vi "Common_Py_Get_Diff_Stats.vi"(0 "session in":refnum<k35>, 5 "module path":path=path "D:/dev/Guy_Storage/Work/Cancun/MW_Display_Test/Magewell Capture/Capture_LV.py", 11 "error in":errorcluster) -> (4 "session out":refnum<k35>, 6 "module path out":path, 14 "Diff_Stats":T1, 15 "error out":errorcluster)   [LabVIEW 2023]
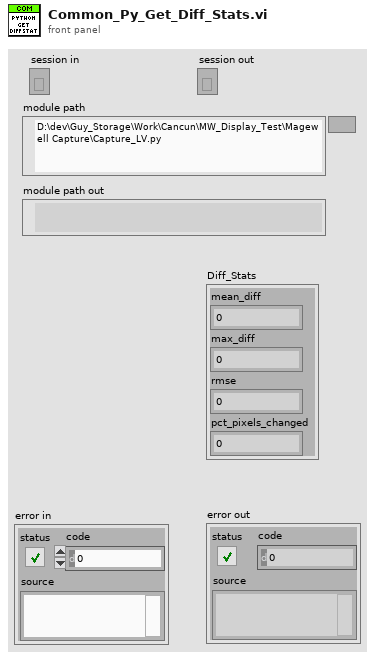
[diagram p1: front panel]
types:
  T1 = cluster{"mean_diff":dbl, "max_diff":dbl, "rmse":dbl, "pct_pixels_changed":dbl}
  T2 = cluster{"[0]":dbl, "[1]":dbl, "[2]":dbl, "[3]":dbl}
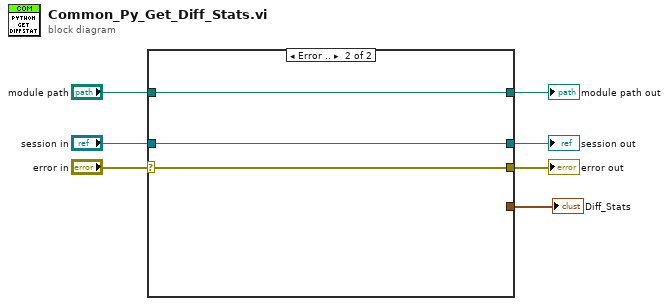
[diagram p0: block diagram]
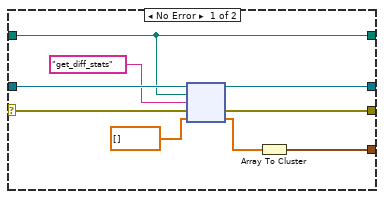
[diagram p2: hidden frame]
diagram:
  n1 = case shown="Error .." "error in" {
    selector: "error in" -> [w13 w18]
    tunnel: "module path" -> [w11 w17]
    tunnel: "session in" -> [w16 w19]
    tunnel: [w15 w18] -> w3
    tunnel: [w14 w19] -> w5
    tunnel: [w11 w17] -> w2
    tunnel: [w8 _] -> w1
    frame No Error {
      n2 = node(w16, w11, "get_diff_stats" ("function name"), w13, dbl[] []) -> (w14:refnum<k35>, w15:errorcluster, w9:dbl[])  [unwired: 2 out]
      n3 = Array To Cluster(array=w9) -> (cluster=w8:T2)
    }
    frame Error {
    }
  }
  "session out" <- w5
  "error out" <- w3
  "module path out" <- w2
  "Diff_Stats" <- w1
